vi "Feedback Nodes.vi"() -> ()   [LabVIEW 2019]
panel:
  in  "Button":bool
  out "Timer":u32
  out "Value in Memory":u32
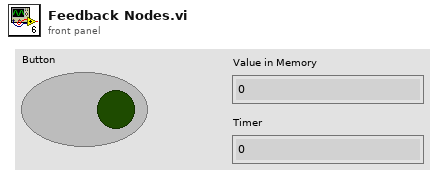
[diagram p1: front panel]
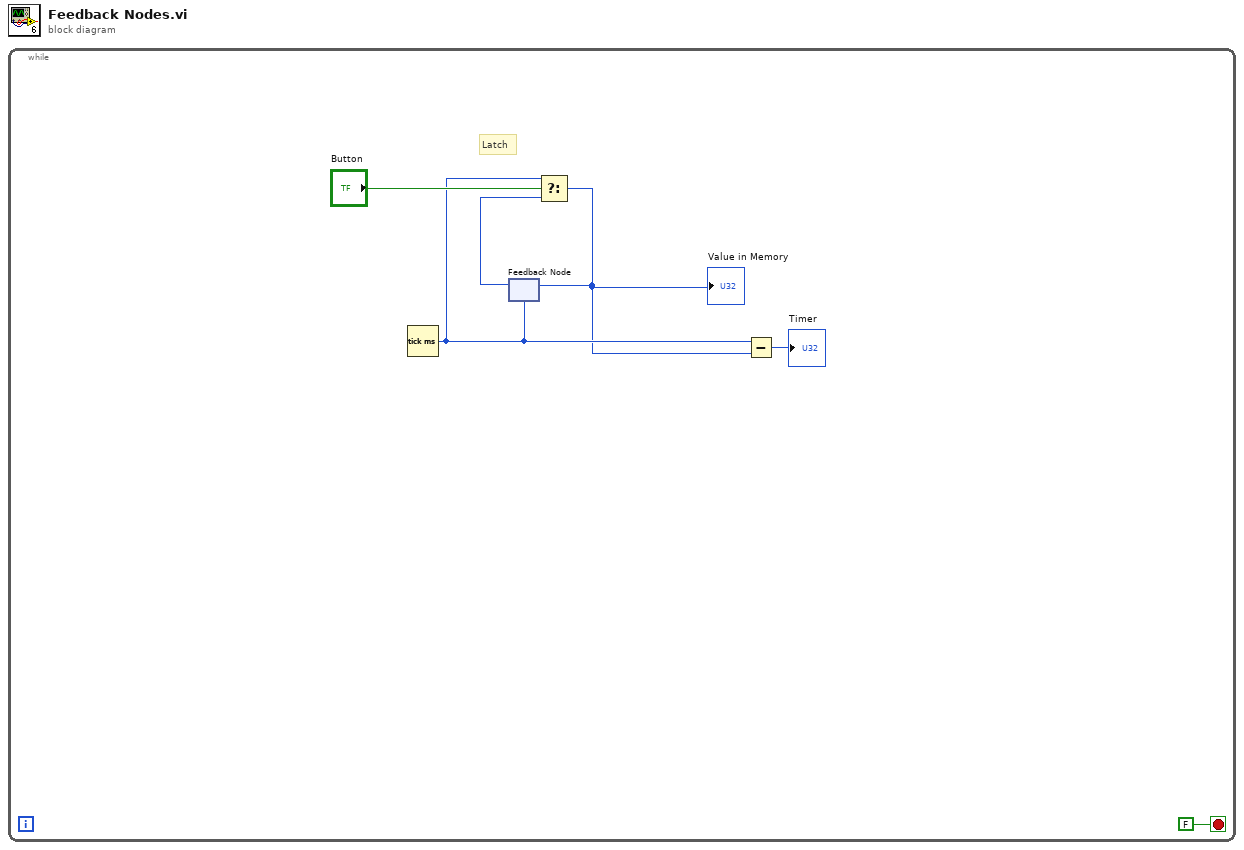
[diagram p0: block diagram]
diagram:
  n1 = while {
    stop <- FALSE stop-if-true
    # "Latch"
    n2 = Tick Count (ms)() -> (millisecond timer value=w3:u32)
    n3 = feedback #1(w3) -> (w2:u32)
    n4 = Select(t=w3, s="Button", f=w2) -> (s? t:f=w1:u32)
    "Value in Memory" <- w1
    n5 = feedback-in #1(w1) -> ()
    n6 = Subtract(x=w3, y=w1) -> (x-y=→"Timer":u32)
  }
